vi "sub UI set Num ref.vi"(8 "error in":errorcluster, 9 "valid":bool, 10 "Value":variant, 11 "num ref":refnum<vi>) -> (0 "error out":errorcluster)   [LabVIEW 2018, in "LF2R IDE.lvlib" / "LF2R IDE.lvclass"]
uses:
  LF2R IDE.lvclass
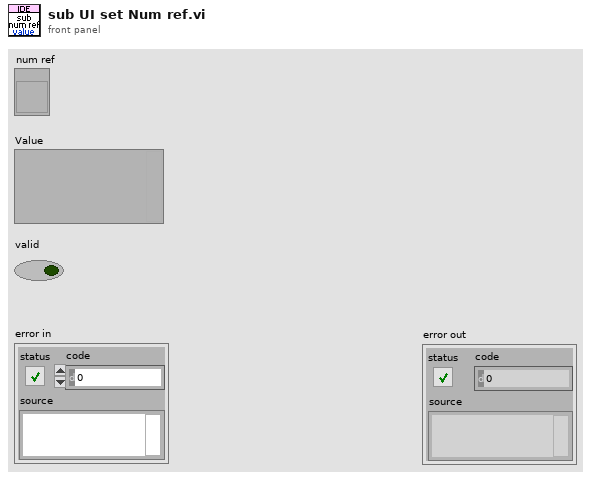
[diagram p1: front panel]
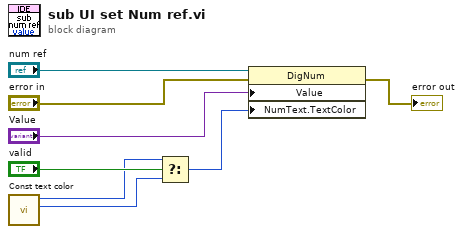
[diagram p0: block diagram]
diagram:
  n1 = call "Const text color.vi"() -> ("invalid num color"=w1:u32, "valid num color"=w2:u32)  [unwired: 10 in]
  n2 = Select(t=w2, s="valid", f=w1) -> (s? t:f=w3:u32)
  n3 = property class="DigNum"(reference="num ref", error in="error in", "Value"="Value", "NumText.TextColor"=w3) -> (error out=→"error out":errorcluster)  [unwired: 1 out]
